vi "Labview and Python.vi"() -> ()   [LabVIEW 2020]
panel:
  out "Input Value":dbl
  out "error in (no error) 3":errorcluster
  out "return value":i32
  in  "error in (no error) 2":errorcluster
  out "error in (no error)":errorcluster
  in  "stop":bool
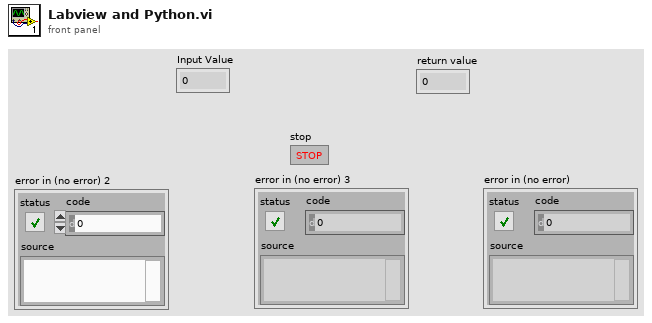
[diagram p1: front panel]
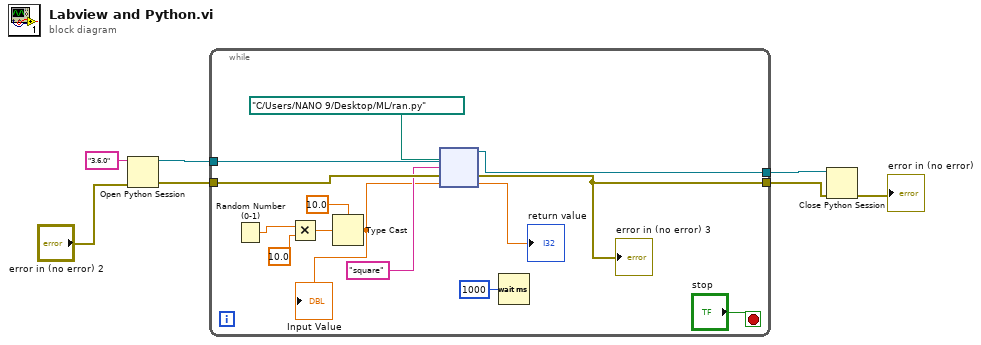
[diagram p0: block diagram]
diagram:
  n1 = Open Python Session(python version="3.6.0" ("Python version"), 3:"error in (no error) 2") -> (session out=w7:refnum<k35>, error out=w4:errorcluster)  [unwired: 1 in]
  n2 = while {
    tunnel: w7 -> [w20]
    tunnel: [w19] -> w6
    tunnel: [w14] -> w5
    tunnel: w4 -> [w18]
    stop <- "stop" stop-if-true
    n3 = Random Number (0-1)() -> (number: 0 to 1=w13:dbl)
    n4 = Multiply(x=w13, y=10.0) -> (x*y=w9:dbl)
    n5 = Type Cast(type=10.0 ("y"), x=w9) -> (*(type *) &x=w10:dbl)
    "Input Value" <- w10
    n6 = node(w20, path "C:/Users/NANO 9/Desktop/ML/ran.py" ("module path"), "square" ("function name"), w18, w10) -> (w19:refnum<k35>, w14:errorcluster, →"return value":dbl)  [unwired: 2 out]
    "error in (no error) 3" <- w14
    n7 = Wait (ms)(milliseconds to wait=u32 1000) -> ()  [unwired: 1 out]
  }
  n8 = Close Python Session(session in=w6, error in=w5) -> (11:→"error in (no error)":errorcluster)
